vi "test Find Disabled Custom Device.vi"(8 "error in":errorcluster, 11 "TestCase in":refnum<class "AIM ARINC 664 EncodeDecode.lvclass">) -> (0 "error out":errorcluster, 3 "TestCase out":refnum<class "AIM ARINC 664 EncodeDecode.lvclass">)   [LabVIEW 2020, in "AIM ARINC 664 EncodeDecode.lvclass"]
uses:
  AIM ARINC 664 EncodeDecode.lvclass
  C:/Program Files (x86)/National Instruments/LabVIEW 2020/vi.lib/NI/VeriStand Custom Device Testing Tools/VeriStandScriptingTestCase/VeriStandScriptingTestCase.lvclass
  <vilib>/NI/VeriStand Custom Device Testing Tools/VeriStandScriptingTestCase/VeriStandScriptingTestCase.lvclass/VeriStandScriptingTestCase.ctl
  <vilib>/NI/VeriStand Custom Device Testing Tools/VeriStandScriptingTestCase/Read Target.vi
  NationalInstruments.VeriStand.SystemDefinitionAPI
  <vilib>/addons/_JKI Toolkits/VI Tester/TestCase.llb/TestCase.lvclass
  Scripting/AIM ARINC 664 Scripting.lvlib
  C:/Program Files (x86)/National Instruments/LabVIEW 2020/vi.lib/addons/_JKI Toolkits/VI Tester/TestCase.llb/TestCase.lvclass
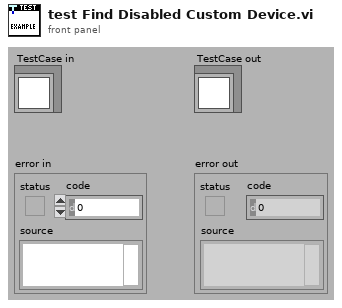
[diagram p1: front panel]
types:
  T1 = typedef "Custom Device API.lvlib/Custom Device Item Ref.ctl" = u64
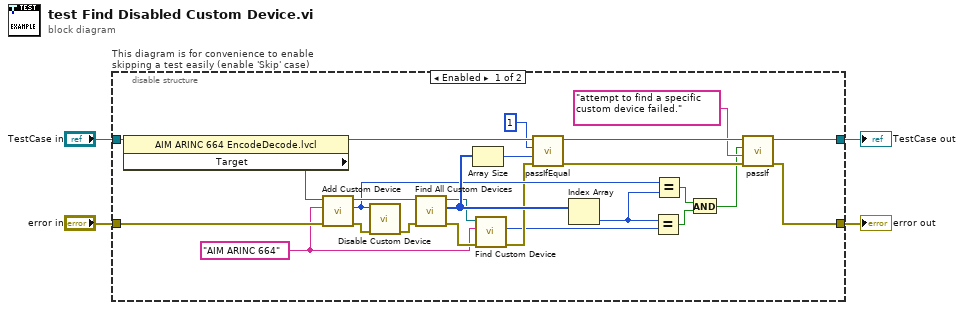
[diagram p0: block diagram]
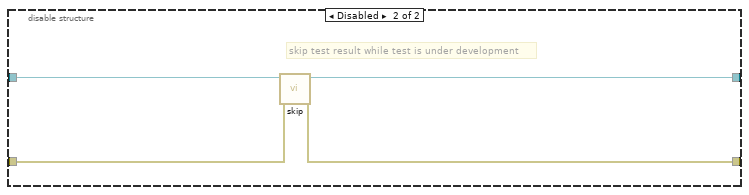
[diagram p2: hidden frame]
diagram:
  n1 = disable-structure "This diagram is for convenience to enable skipping a test easily (enable 'Skip' case)" shown="Enabled" {
    disable-tunnel: "TestCase in" -> [w26 w33]
    disable-tunnel: [w25 w31] -> w1
    disable-tunnel: [w24 w32] -> w3
    disable-tunnel: "error in" -> [w29 w30]
    frame Enabled {
      w5 = "AIM ARINC 664" ("name")
      n2 = property class="AIM ARINC 664 EncodeDecode.lvcl"(reference=w26) -> (reference out=w28:refnum<class "AIM ARINC 664 EncodeDecode.lvclass">, "Target"=w23:refnum<k24>)  [unwired: 1 in, 1 out]
      n3 = call "Add Custom Device.vi"("error in"=w29, "name"=w5, "target in"=w23) -> ("error out"=w22:errorcluster, "custom device"=w10:T1, "target out"=w12:refnum<k24>)  [unwired: 6 in]
      n4 = call "Disable Custom Device.vi"("error in"=w22, "custom device ref in"=w10) -> ("error out"=w20:errorcluster)  [unwired: 8 in, 1 out]
      n5 = call "Find All Custom Devices.vi"("error in"=w20, "target in"=w12) -> ("error out"=w21:errorcluster, "custom devices"=w11:u64[], "target out"=w6:refnum<k24>)  [unwired: 7 in]
      n6 = Array Size(array=w11) -> (size(s)=w13:i32)
      n7 = call "Find Custom Device.vi"("error in"=w21, "name"=w5, "target in"=w6) -> ("error out"=w8:errorcluster, "custom device"=w7:u64)  [unwired: 6 in, 1 out]
      n8 = call-dynamic "passIfEqual.vi"("error in (no error)"=w8, "y"=w13, "x"=1 ("disabled custom device"), "TestCase in"=w28) -> ("error out"=w19:errorcluster, "TestCase out"=w27:refnum<class "AIM ARINC 664 EncodeDecode.lvclass">)  [unwired: 6 in]
      n9 = Index Array(array=w11) -> (element=w9:u64)  [unwired: 1 in]
      n10 = Equal?(x=w9, y=w7) -> (x = y?=w18:bool)
      n11 = Equal?(x=w10, y=w9) -> (x = y?=w17:bool)
      n12 = And(x=w17, y=w18) -> (x .and. y?=w15:bool)
      n13 = call-dynamic "passIf.vi"("error in (no error)"=w19, "message (\"\")"="attempt to find a specific custom device failed." ("message (\"\")"), "pass"=w15, "TestCase in"=w27) -> ("error out"=w24:errorcluster, "TestCase out"=w25:refnum<class "AIM ARINC 664 EncodeDecode.lvclass">)  [unwired: 6 in]
    }
    frame Disabled {
      # "skip test result while test is under development"
      n14 = call <vilib>:"skip.vi"("error in (no error)"=w30, "TestCase in"=w33) -> ("error out"=w32:errorcluster, "TestCase out"=w31:refnum<class "AIM ARINC 664 EncodeDecode.lvclass">)  [unwired: 8 in]
    }
  }
  "error out" <- w3
  "TestCase out" <- w1
